vi "test-traj-generate-1-way.vi"() -> ()   [LabVIEW 2019]
uses:
  <vilib>/Rock Robotics/WPI/ThirdParty/JAS_Junk/TrajLib/TRAJ_CONFIG.ctl
  <vilib>/Rock Robotics/WPI/ThirdParty/JAS_Junk/TrajLib/TRAJ_CONSTRAINT_DIIF_DRIVE_KINEMATICS.ctl
  <vilib>/Rock Robotics/WPI/ThirdParty/JAS_Junk/TrajLib/DIFF_DRIVE_KINEMATICS.ctl
  <vilib>/Rock Robotics/WPI/ThirdParty/JAS_Junk/TrajLib/TRAJ_CONSTRAINT_CENTRIPETAL_ACCEL.ctl
  <vilib>/Rock Robotics/WPI/ThirdParty/JAS_Junk/TrajLib/TRAJ_CONSTRAINT_SWERVE_DRIVE_KINEMATICS.ctl
  <vilib>/Rock Robotics/WPI/ThirdParty/JAS_Junk/TrajLib/SWERVE_DRIVE_KINEMATICS.ctl
  <vilib>/Analysis/Matrix/Datatypes/RealMatrix.ctl
  <vilib>/Rock Robotics/WPI/ThirdParty/JAS_Junk/TrajLib/TRANSLATION2D.ctl
  <vilib>/Rock Robotics/WPI/ThirdParty/JAS_Junk/TrajLib/TRAJ_CONSTRAINT_DIIF_DRIVE_VOLTAGE.ctl
  <vilib>/Rock Robotics/WPI/ThirdParty/JAS_Junk/TrajLib/SIMPLE_MOTOR_FF.ctl
  <vilib>/Rock Robotics/WPI/ThirdParty/JAS_Junk/TrajLib/TRAJ_CONSTRAINT_MECA_DRIVE_KINEMATICS.ctl
  <vilib>/Rock Robotics/WPI/ThirdParty/JAS_Junk/TrajLib/MECA_DRIVE_KINEMATICS.ctl
  <vilib>/Rock Robotics/WPI/ThirdParty/JAS_Junk/TrajLib/TRAJECTORY.ctl
  <vilib>/Rock Robotics/WPI/ThirdParty/JAS_Junk/TrajLib/TRAJ_STATE.ctl
  <vilib>/Rock Robotics/WPI/ThirdParty/JAS_Junk/TrajLib/POSE2D.ctl
  <vilib>/Rock Robotics/WPI/ThirdParty/JAS_Junk/TrajLib/ROTATION2D.ctl
  <vilib>/Rock Robotics/WPI/ThirdParty/JAS_Junk/TrajLib/UTIL_WAYPOINT.ctl
  <vilib>/Rock Robotics/WPI/ThirdParty/JAS_Junk/TrajLib/SPLINE.ctl
  <vilib>/Rock Robotics/WPI/ThirdParty/JAS_Junk/TrajLib/POSEwCURVATURE.ctl
  <vilib>/Rock Robotics/WPI/ThirdParty/JAS_Junk/TrajLib/SPLINE_CTRL_VECTOR.ctl
  <vilib>/Rock Robotics/WPI/ThirdParty/JAS_Junk/TrajLib/Rotation_CreateAngle.vi
  <vilib>/Rock Robotics/WPI/ThirdParty/JAS_Junk/TrajLib/Translation_Create.vi
  <vilib>/Rock Robotics/WPI/ThirdParty/JAS_Junk/TrajLib/Trajectory_Library.lvlib
  <vilib>/Analysis/Matrix/NI_Matrix.lvlib
panel:
  in  "Tab Control":T1(tab)
  in  "Initial_Position":T2={"X"=0.0, "Y"=-2.0, "ANGLE"=0.0} {"ANGLE" format="%13.3f"; "Y" format="%13.3f"; "X" format="%13.3f"}
  in  "Ending_Position":T2={"X"=2.0, "Y"=0.0, "ANGLE"=1.57} {"ANGLE" format="%13.3f"; "Y" format="%13.3f"; "X" format="%13.3f"}
  out "initialSpline_Ctrl_Vector":T3
  out "endSpline_Ctrl_Vector":T3
  in  "Interior WAYPOINTS":T4[](array[typedef])=[{"X"=1.414, "Y"=-1.414}] {"Y" format="%14.3f"; "X" format="%14.3f"}
  out "splines":T5[](array[typedef])
  out "ArrayPoseWithCurvature":T7[](array[typedef])
  out "PoseCSize":i32
  out "error out 2":errorcluster
  in  "Config":T10={"MaxVelocity"=2.0, "Max Acceleration"=2.0, "StartVelocity"=0.0, "End Velocity"=0.0, "Reversed"=FALSE, "DiffDrKineConstntDefined"=FALSE, "CentAcellConstntDefined"=FALSE, "DiffDrVoltConstntDefined"=FALSE, "DIFF_DRIVE_KINE_CONSTRAINT"={"Max Speed (M/S)"=0.0, "DIFF_DRIVE_KINEMATICS"={"TrackWidth_Meters"=0.0}}, "CENTRIPETAL_ACCEL_CONSTRAINT"={"Max Cent Accel"=0.0}, "SwerveDrKineConstntDefined"=FALSE, "SWERVE_DRIVE_KINE_CONSTRAINT"={"Max Speed (M/S)"=0.0, "SwerveKinematics"={"NumModules"=0, "InverseKinematics"=[], "ForwardKinematics"=[], "Modules"=[], "PrevCoR"={"X"=0.0, "Y"=0.0}}}, "DIFF_DRIVE_VOLTAGE_CONSTRAINT"={"Max Voltage"=0.0, "DIFF_DRIVE_KINEMATICS"={"TrackWidth_Meters"=0.0}, "SIMPLE_MOTOR_FF"={"Ks"=0.0, "Kv"=0.0, "Ka"=0.0}}, "MECANUM_DRIVE_KINE_CONSTRAINT"={"Max Speed (M/S)"=0.0, "MECA_DRIVE_KINEMATICS"={"FrontLeft"={"X"=0.0, "Y"=0.0}, "FrontRight"={"X"=0.0, "Y"=0.0}, "RearLeft"={"X"=0.0, "Y"=0.0}, "RearRight"={"X"=0.0, "Y"=0.0}, "InverseKinematics"=[[0.0, 1.0, -1.0, 0.0], [0.0, 1.0, 1.0, 0.0], [0.0, 1.0, 1.0, 0.0], [0.0, 1.0, -1.0, 0.0]], "ForwardKinematics"=[[0.0, 1.0, -1.0, 0.0], [0.0, 1.0, 1.0, 0.0], [0.0, 1.0, 1.0, 0.0], [0.0, 1.0, -1.0, 0.0]], "PrevCoR"={"X"=0.0, "Y"=0.0}}}, "MecanumDrKineConstntDefined"=FALSE} {"MECANUM_DRIVE_KINE_CONSTRAINT"."MECA_DRIVE_KINEMATICS"."PrevCoR"."Y" format="%14.3f"; "MECANUM_DRIVE_KINE_CONSTRAINT"."MECA_DRIVE_KINEMATICS"."PrevCoR"."X" format="%14.3f"; "MECANUM_DRIVE_KINE_CONSTRAINT"."MECA_DRIVE_KINEMATICS"."RearRight"."Y" format="%14.3f"; "MECANUM_DRIVE_KINE_CONSTRAINT"."MECA_DRIVE_KINEMATICS"."RearRight"."X" format="%14.3f"; "MECANUM_DRIVE_KINE_CONSTRAINT"."MECA_DRIVE_KINEMATICS"."RearLeft"."Y" format="%14.3f"; "MECANUM_DRIVE_KINE_CONSTRAINT"."MECA_DRIVE_KINEMATICS"."RearLeft"."X" format="%14.3f"; "MECANUM_DRIVE_KINE_CONSTRAINT"."MECA_DRIVE_KINEMATICS"."FrontRight"."Y" format="%14.3f"; "MECANUM_DRIVE_KINE_CONSTRAINT"."MECA_DRIVE_KINEMATICS"."FrontRight"."X" format="%14.3f"; "MECANUM_DRIVE_KINE_CONSTRAINT"."MECA_DRIVE_KINEMATICS"."FrontLeft"."Y" format="%14.3f"; "MECANUM_DRIVE_KINE_CONSTRAINT"."MECA_DRIVE_KINEMATICS"."FrontLeft"."X" format="%14.3f"; "MECANUM_DRIVE_KINE_CONSTRAINT"."Max Speed (M/S)" format="%20.4f"; "DIFF_DRIVE_VOLTAGE_CONSTRAINT"."SIMPLE_MOTOR_FF"."Ka" format="%13.4f"; "DIFF_DRIVE_VOLTAGE_CONSTRAINT"."SIMPLE_MOTOR_FF"."Kv" format="%13.4f"; "DIFF_DRIVE_VOLTAGE_CONSTRAINT"."SIMPLE_MOTOR_FF"."Ks" format="%13.4f"; "DIFF_DRIVE_VOLTAGE_CONSTRAINT"."DIFF_DRIVE_KINEMATICS"."TrackWidth_Meters" format="%20.4f"; "DIFF_DRIVE_VOLTAGE_CONSTRAINT"."Max Voltage" format="%20.4f"; "SWERVE_DRIVE_KINE_CONSTRAINT"."SwerveKinematics"."PrevCoR"."Y" format="%14.3f"; "SWERVE_DRIVE_KINE_CONSTRAINT"."SwerveKinematics"."PrevCoR"."X" format="%14.3f"; "SWERVE_DRIVE_KINE_CONSTRAINT"."SwerveKinematics"."Modules"."Y" format="%14.3f"; "SWERVE_DRIVE_KINE_CONSTRAINT"."SwerveKinematics"."Modules"."X" format="%14.3f"; "SWERVE_DRIVE_KINE_CONSTRAINT"."Max Speed (M/S)" format="%20.4f"; "CENTRIPETAL_ACCEL_CONSTRAINT"."Max Cent Accel" format="%20.4f"; "DIFF_DRIVE_KINE_CONSTRAINT"."DIFF_DRIVE_KINEMATICS"."TrackWidth_Meters" format="%20.4f"; "DIFF_DRIVE_KINE_CONSTRAINT"."Max Speed (M/S)" format="%20.4f"; "End Velocity" format="%20.4f"; "StartVelocity" format="%20.4f"; "Max Acceleration" format="%20.4f"; "MaxVelocity" format="%20.4f"}
  out "TRAJECTORY":T20 {"TotalTImeSecs" format="%20.3f"}
  out "size(s)":i32
  out "error out":errorcluster
  out "XY Graph":cluster{dbl[], dbl[]}(graph)
  out "Position":cluster{dbl[], dbl[]}(graph)
  out "Done":bool
  # "ARRAY OF OTHER\nCONSTRAINTS \nGOES HERE.."
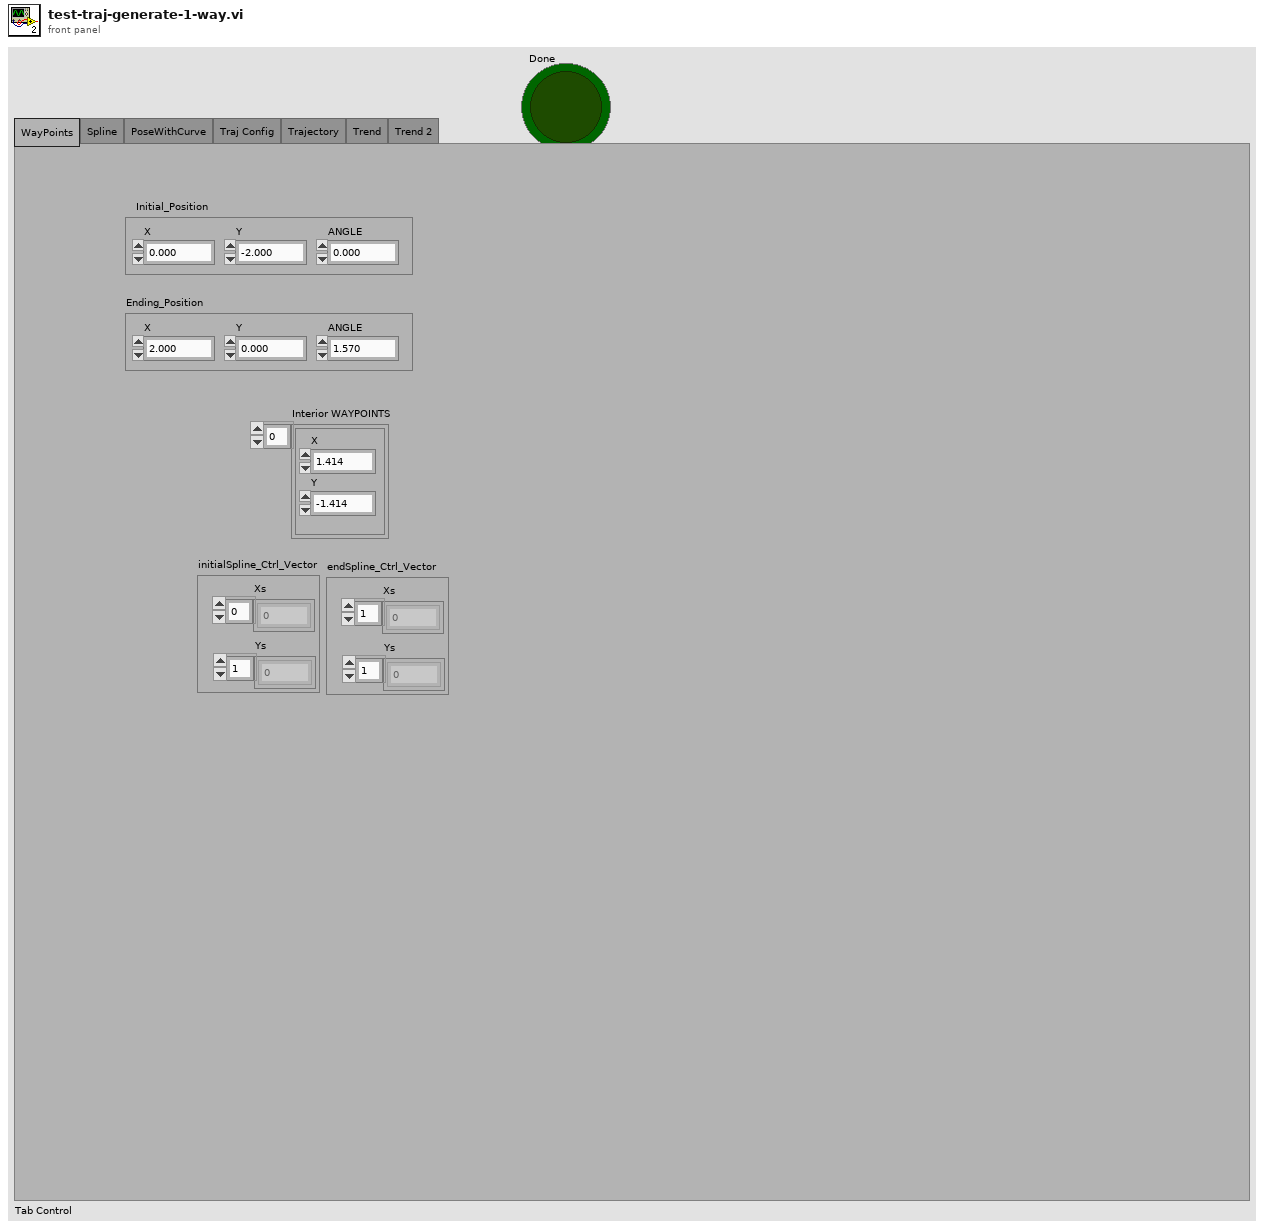
[diagram p1: front panel]
types:
  T1 = enum32{"WayPoints", "Spline", "PoseWithCurve", "Traj Config", "Trajectory", "Trend", "Trend 2"}
  T2 = typedef "Trajectory_Library.lvlib/UTIL_WAYPOINT.ctl" = cluster{"X":dbl, "Y":dbl, "ANGLE":dbl}
  T3 = typedef "Trajectory_Library.lvlib/SPLINE_CTRL_VECTOR.ctl" = cluster{"Xs":dbl[], "Ys":dbl[]}
  T4 = typedef "Trajectory_Library.lvlib/TRANSLATION2D.ctl" = cluster{"X":dbl, "Y":dbl}
  T5 = typedef "Trajectory_Library.lvlib/SPLINE.ctl" = cluster{"Degree":i32, "Coefficients":T6}
  T6 = typedef "NI_Matrix.lvlib/RealMatrix.ctl" = dbl[][]
  T7 = typedef "Trajectory_Library.lvlib/POSEwCURVATURE.ctl" = cluster{"CURVATURE":dbl, "POSE":T8}
  T8 = typedef "Trajectory_Library.lvlib/POSE2D.ctl" = cluster{"TRANSLATION":T4, "ROTATION":T9}
  T9 = typedef "Trajectory_Library.lvlib/ROTATION2D.ctl" = cluster{"VALUE":dbl, "COS":dbl, "SIN":dbl}
  T10 = typedef "Trajectory_Library.lvlib/TRAJ_CONFIG.ctl" = cluster{"MaxVelocity":dbl, "Max Acceleration":dbl, "StartVelocity":dbl, "End Velocity":dbl, "Reversed":bool, "DiffDrKineConstntDefined":bool, "CentAcellConstntDefined":bool, "DiffDrVoltConstntDefined":bool, "DIFF_DRIVE_KINE_CONSTRAINT":T11, "CENTRIPETAL_ACCEL_CONSTRAINT":T13, "SwerveDrKineConstntDefined":bool, "SWERVE_DRIVE_KINE_CONSTRAINT":T14, "DIFF_DRIVE_VOLTAGE_CONSTRAINT":T16, "MECANUM_DRIVE_KINE_CONSTRAINT":T18, "MecanumDrKineConstntDefined":bool}
  T11 = typedef "Trajectory_Library.lvlib/TRAJ_CONSTRAINT_DIIF_DRIVE_KINEMATICS.ctl" = cluster{"Max Speed (M/S)":dbl, "DIFF_DRIVE_KINEMATICS":T12}
  T12 = typedef "Trajectory_Library.lvlib/DIFF_DRIVE_KINEMATICS.ctl" = cluster{"TrackWidth_Meters":dbl}
  T13 = typedef "Trajectory_Library.lvlib/TRAJ_CONSTRAINT_CENTRIPETAL_ACCEL.ctl" = cluster{"Max Cent Accel":dbl}
  T14 = typedef "Trajectory_Library.lvlib/TRAJ_CONSTRAINT_SWERVE_DRIVE_KINEMATICS.ctl" = cluster{"Max Speed (M/S)":dbl, "SwerveKinematics":T15}
  T15 = typedef "Trajectory_Library.lvlib/SWERVE_DRIVE_KINEMATICS.ctl" = cluster{"NumModules":i32, "InverseKinematics":T6, "ForwardKinematics":T6, "Modules":T4[], "PrevCoR":T4}
  T16 = typedef "Trajectory_Library.lvlib/TRAJ_CONSTRAINT_DIIF_DRIVE_VOLTAGE.ctl" = cluster{"Max Voltage":dbl, "DIFF_DRIVE_KINEMATICS":T12, "SIMPLE_MOTOR_FF":T17}
  T17 = typedef "Trajectory_Library.lvlib/SIMPLE_MOTOR_FF.ctl" = cluster{"Ks":dbl, "Kv":dbl, "Ka":dbl}
  T18 = typedef "Trajectory_Library.lvlib/TRAJ_CONSTRAINT_MECA_DRIVE_KINEMATICS.ctl" = cluster{"Max Speed (M/S)":dbl, "MECA_DRIVE_KINEMATICS":T19}
  T19 = typedef "Trajectory_Library.lvlib/MECA_DRIVE_KINEMATICS.ctl" = cluster{"FrontLeft":T4, "FrontRight":T4, "RearLeft":T4, "RearRight":T4, "InverseKinematics":T6, "ForwardKinematics":T6, "PrevCoR":T4}
  T20 = typedef "Trajectory_Library.lvlib/TRAJECTORY.ctl" = cluster{"TotalTImeSecs":dbl, "States":T21[]}
  T21 = typedef "Trajectory_Library.lvlib/TRAJ_STATE.ctl" = cluster{"TimeSeconds":dbl, "Velocity":dbl, "Acceleration":dbl, "POSE":T8, "Curvature":dbl}
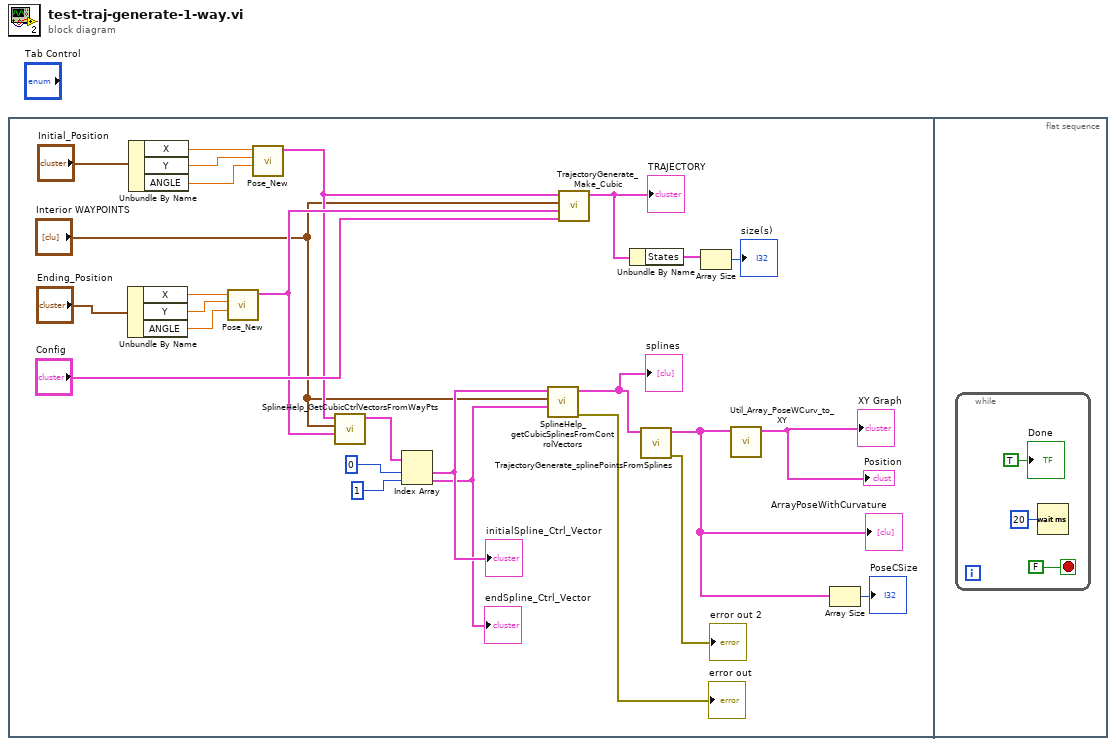
[diagram p0: block diagram]
diagram:
  n1 = flat-sequence {
    frame #0 {
      n2 = Unbundle By Name("Ending_Position") -> ("X"=w21:dbl, "Y"=w20:dbl, "ANGLE"=w19:dbl)
      n3 = Unbundle By Name("Initial_Position") -> ("X"=w24:dbl, "Y"=w23:dbl, "ANGLE"=w22:dbl)
      n4 = call <vilib>:"Pose_New.vi"("Heading"=w19, "Y"=w20, "X"=w21) -> ("out POSe"=w17:T8)  [unwired: 8 in]
      n5 = call <vilib>:"Pose_New.vi"("Heading"=w22, "Y"=w23, "X"=w24) -> ("out POSe"=w16:T8)  [unwired: 8 in]
      n6 = call <vilib>:"SplineHelp_GetCubicCtrlVectorsFromWayPts.vi"("Enging POSE"=w17, "Interior WAYPOINTS"="Interior WAYPOINTS", "Starting POSE"=w16) -> ("SplineControlVectors"=w5:T3[])  [unwired: 8 in]
      n7 = Index Array(array=w5, index #1=0 ("index"), index #2=1 ("index")) -> (element #1=w4:T3, element #2=w3:T3)
      "initialSpline_Ctrl_Vector" <- w4
      "endSpline_Ctrl_Vector" <- w3
      n8 = call <vilib>:"SplineHelp_getCubicSplinesFromControlVectors.vi"("endCtrlVector"=w3, "InternalWaypoints"="Interior WAYPOINTS", "startCtrlVector"=w4) -> ("error out"=→"error out":errorcluster, "splines"=w15:T5[])  [unwired: 3 in, 4 out]
      "splines" <- w15
      n9 = call <vilib>:"TrajectoryGenerate_Make_Cubic.vi"("traj_config"="Config", "Enging POSE"=w17, "Interior WAYPOINTS"="Interior WAYPOINTS", "Starting POSE"=w16) -> ("TRAJECTORY"=w13:T20)  [unwired: 6 in, 1 out]
      "TRAJECTORY" <- w13
      n10 = Unbundle By Name(w13) -> ("States"=w12:T21[])
      n11 = call <vilib>:"TrajectoryGenerate_splinePointsFromSplines.vi"("inputSPLINE"=w15) -> ("error out"=→"error out 2":errorcluster, "ArrayPoseWithCurvature"=w9:T7[])  [unwired: 9 in]
      "ArrayPoseWithCurvature" <- w9
      n12 = Array Size(array=w12) -> (size(s)=→"size(s)":i32)
      n13 = call <vilib>:"Util_Array_PoseWCurv_to_XY.vi"("inArrayPoseWCurve"=w9) -> ("outArrayXY"=→"XY Graph" →"Position":cluster{dbl[], dbl[]})  [unwired: 10 in]
      n14 = Array Size(array=w9) -> (size(s)=→"PoseCSize":i32)
    }
    frame #1 {
      n15 = while {
        stop <- FALSE stop-if-true
        n16 = Wait (ms)(milliseconds to wait=u32 20) -> ()  [unwired: 1 out]
        "Done" <- TRUE ("Done")
      }
    }
  }
